vi "sub_selector.vi"(9 "波形":T1, 10 "数组":waveform(dbl)[](array[waveform]), 11 "布尔":bool) -> (3 "波形输出UI 7":T4)   [LabVIEW 2018, in "UI.lvlib"]
uses:
  UI.lvlib
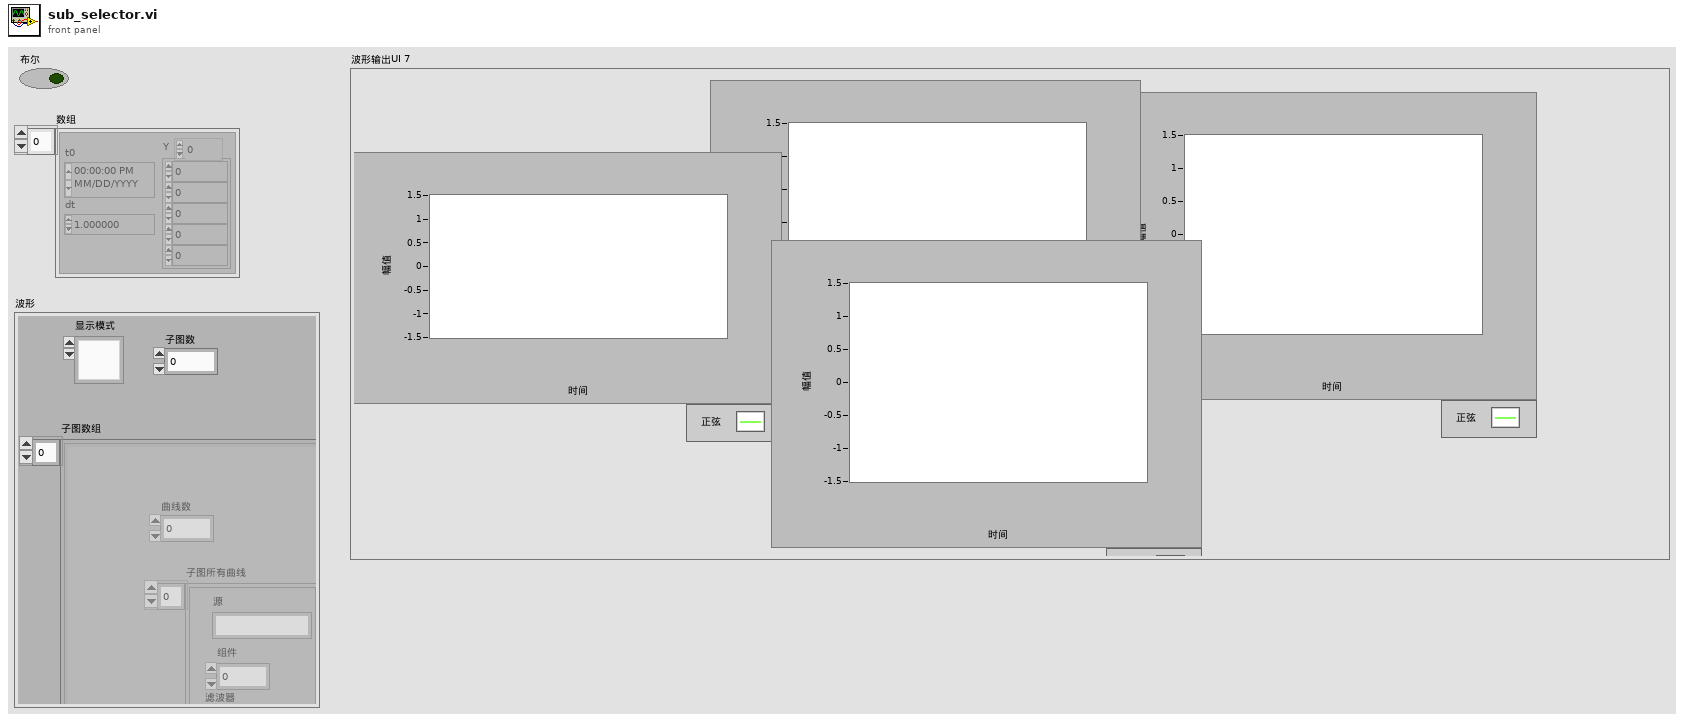
[diagram p1: front panel]
types:
  T1 = typedef "波形图.ctl" = cluster{"显示模式":u16, "子图数":u32, "子图数组":T2[]}
  T2 = typedef "子图.ctl" = cluster{"子图所有曲线":T3[], "曲线数":u32}
  T3 = typedef "曲线簇.ctl" = cluster{"源":string, "组件":u32, "滤波器":u32}
  T4 = typedef "控件 13.ctl" = cluster{"数据 1":waveform(dbl)[], "数据 2":waveform(dbl)[], "数据 3":waveform(dbl)[], "数据 4":waveform(dbl)[]}
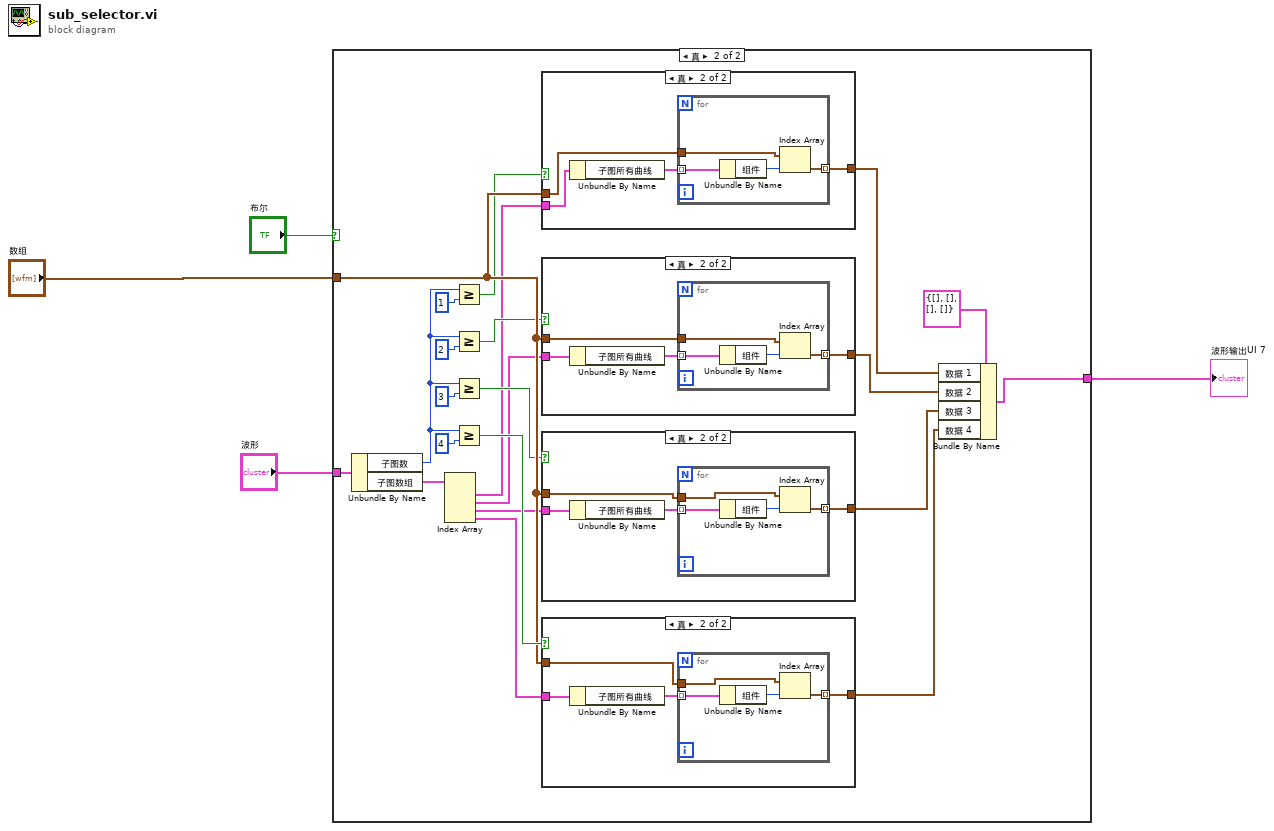
[diagram p0: block diagram]
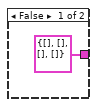
[diagram p2: hidden frame]
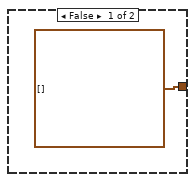
[diagram p3: hidden frame]
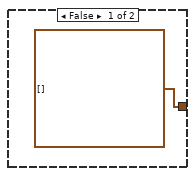
[diagram p4: hidden frame]
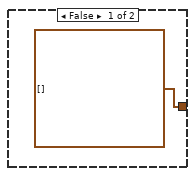
[diagram p5: hidden frame]
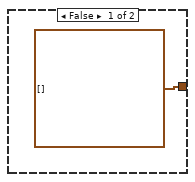
[diagram p6: hidden frame]
diagram:
  n1 = case shown="真" "布尔" {
    tunnel: "波形" -> [_ w27]
    tunnel: "数组" -> [_ w23]
    tunnel: [T4 {"数据 1"=[], "数据 2"=[], "数据 3"=[], "数据 4"=[]} ("波形输出UI 7") w7] -> w4
    frame False {
    }
    frame True {
      n2 = Unbundle By Name(w27) -> ("子图数"=w16:u32, "子图数组"=w24:T2[])
      n3 = Index Array(array=w24) -> (element #1=w11:T2, element #2=w10:T2, element #3=w9:T2, element #4=w8:T2)  [unwired: 4 in]
      n4 = Greater Or Equal?(x=w16, y=1) -> (x >= y?=w17:bool)
      n5 = Greater Or Equal?(x=w16, y=2) -> (x >= y?=w18:bool)
      n6 = Greater Or Equal?(x=w16, y=3) -> (x >= y?=w19:bool)
      n7 = Greater Or Equal?(x=w16, y=4) -> (x >= y?=w26:bool)
      n8 = case shown="真" w17 {
        tunnel: w23 -> [_ w49]
        tunnel: [waveform(dbl)[] [] w47] -> w12
        tunnel: w11 -> [_ w48]
        frame False {
        }
        frame True {
          n9 = Unbundle By Name(w48) -> ("子图所有曲线"=w50:T3[])
          n10 = for {
            tunnel: w50 -> [w54] mode=indexing
            tunnel: w49 -> [w53]
            tunnel: [w51] -> w47 mode=indexing
            n11 = Unbundle By Name(w54) -> ("组件"=w52:u32)
            n12 = Index Array(array=w53, index=w52) -> (element=w51:waveform(dbl))
          }
        }
      }
      n13 = case shown="真" w18 {
        tunnel: w23 -> [_ w40]
        tunnel: [waveform(dbl)[] [] w38] -> w13
        tunnel: w10 -> [_ w39]
        frame False {
        }
        frame True {
          n14 = Unbundle By Name(w39) -> ("子图所有曲线"=w41:T3[])
          n15 = for {
            tunnel: w41 -> [w45] mode=indexing
            tunnel: w40 -> [w43]
            tunnel: [w42] -> w38 mode=indexing
            n16 = Unbundle By Name(w45) -> ("组件"=w44:u32)
            n17 = Index Array(array=w43, index=w44) -> (element=w42:waveform(dbl))
          }
        }
      }
      n18 = case shown="真" w19 {
        tunnel: w9 -> [_ w32]
        tunnel: w23 -> [_ w30]
        tunnel: [waveform(dbl)[] [] w29] -> w14
        frame False {
        }
        frame True {
          n19 = Unbundle By Name(w32) -> ("子图所有曲线"=w31:T3[])
          n20 = for {
            tunnel: w31 -> [w36] mode=indexing
            tunnel: w30 -> [w34]
            tunnel: [w33] -> w29 mode=indexing
            n21 = Unbundle By Name(w36) -> ("组件"=w35:u32)
            n22 = Index Array(array=w34, index=w35) -> (element=w33:waveform(dbl))
          }
        }
      }
      n23 = case shown="真" w26 {
        tunnel: w23 -> [_ w58]
        tunnel: [waveform(dbl)[] [] w57] -> w15
        tunnel: w8 -> [_ w56]
        frame False {
        }
        frame True {
          n24 = Unbundle By Name(w56) -> ("子图所有曲线"=w59:T3[])
          n25 = for {
            tunnel: w59 -> [w63] mode=indexing
            tunnel: w58 -> [w62]
            tunnel: [w60] -> w57 mode=indexing
            n26 = Unbundle By Name(w63) -> ("组件"=w61:u32)
            n27 = Index Array(array=w62, index=w61) -> (element=w60:waveform(dbl))
          }
        }
      }
      n28 = Bundle By Name(cluster=T4 {"数据 1"=[], "数据 2"=[], "数据 3"=[], "数据 4"=[]} ("波形输出UI 7"), "数据 1"=w12, "数据 2"=w13, "数据 3"=w14, "数据 4"=w15) -> (w7:T4)
    }
  }
  "波形输出UI 7" <- w4
